vi "Auto-Pause Check.vi"(6 "Auto Stats":T1, 10 "Queue":refnum<queue>, 11 "Autopause":cluster{"GoodPause":u32, "RejectPause":u32}) -> (3 "Autopause out":cluster{"GoodPause":u32, "RejectPause":u32})   [LabVIEW 2021]
uses:
  support/Controls/Auto Stats.ctl
  RT/Controls/Auto Times.ctl
  support/Message Queue/Message Cluster.ctl
  support/Message Queue/Enqueue Message (Single).vi
  <vilib>/ErrorRing/Error Ring.xnode
  support/Message Queue/Message Queue.lvlib
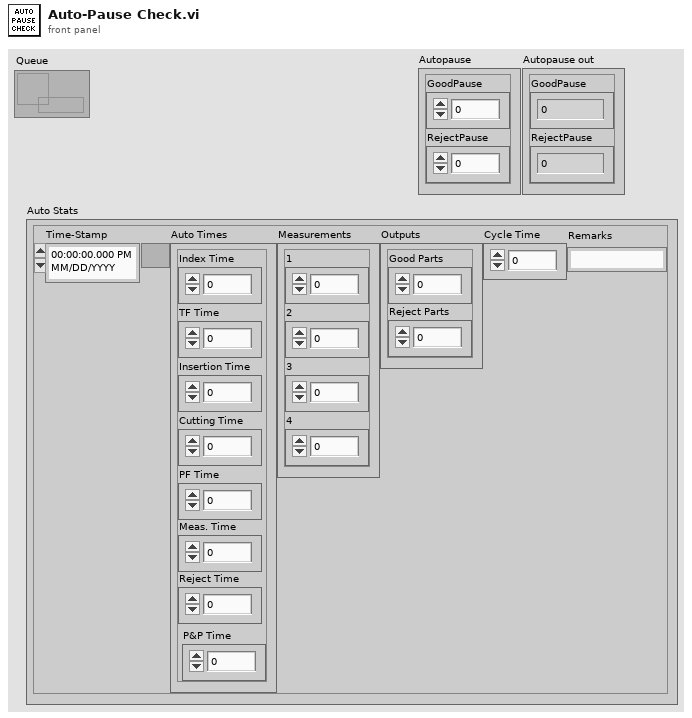
[diagram p1: front panel]
types:
  T1 = typedef "Auto Stats.ctl" = cluster{"Time-Stamp":timestamp, "Auto Times":T2, "Measurements":cluster{"1":dbl, "2":dbl, "3":dbl, "4":dbl}, "Outputs":cluster{"Good Parts":u32, "Reject Parts":u32}, "Cycle Time":dbl, "Remarks":string}
  T2 = typedef "Auto Times.ctl" = cluster{"Index Time":u32, "TF Time":u32, "Insertion Time":u32, "Cutting Time":u32, "PF Time":u32, "Meas. Time":u32, "Reject Time":u32, "P&P Time":u32}
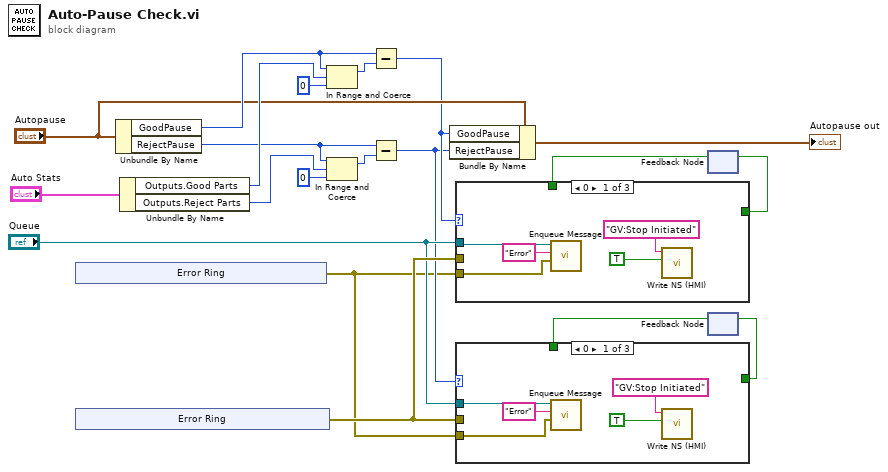
[diagram p0: block diagram]
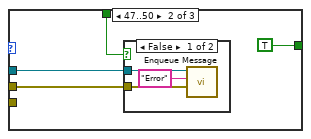
[diagram p2: hidden frame]
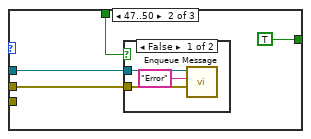
[diagram p5: hidden frame]
diagram:
  n1 = xnode "Error Ring"() -> ("error out"=w1:errorcluster)
  n2 = xnode "Error Ring"() -> ("error out"=w14:errorcluster)
  n3 = Unbundle By Name("Autopause") -> ("GoodPause"=w19:u32, "RejectPause"=w7:u32)
  n4 = Unbundle By Name("Auto Stats") -> ("Outputs.Good Parts"=w18:u32, "Outputs.Reject Parts"=w8:u32)
  n5 = In Range and Coerce(upper limit=w19, x=w18, lower limit=u32 0) -> (coerced(x)=w11:u32)  [unwired: 1 out]
  n6 = In Range and Coerce(upper limit=w7, x=w8, lower limit=u32 0) -> (coerced(x)=w10:u32)  [unwired: 1 out]
  n7 = Subtract(x=w19, y=w11) -> (x-y=w15:u32)
  n8 = Subtract(x=w7, y=w10) -> (x-y=w6:u32)
  n9 = Bundle By Name(cluster="Autopause", "GoodPause"=w15, "RejectPause"=w6) -> (→"Autopause out":cluster{"GoodPause":u32, "RejectPause":u32})
  n10 = feedback #1() -> (w4:bool)  [unwired: 1 in]
  n11 = case shown="0" w15 {
    tunnel: "Queue" -> [w22 w29 _]
    tunnel: w14 -> [_ w28 _]
    tunnel: [_ TRUE _] -> w5
    tunnel: w4 -> [_ w26 _]
    tunnel: w1 -> [w21 _ _]
    frame 0 {
      n12 = call-poly "Enqueue Message.vi"("Message Data"=w21, "Message"="Error", "Message Queue"=w22) -> ()  [unwired: 7 in, 2 out]
      n13 = call "Write NS (HMI).vi"("Message Data"=TRUE, "Message"="GV:Stop Initiated" ("string")) -> ()  [unwired: 9 in, 1 out]
    }
    frame 47..50 {
      n14 = case shown="False" w26 {
        tunnel: w29 -> [w31 _]
        tunnel: w28 -> [w30 _]
        frame False {
          n15 = call-poly "Enqueue Message.vi"("Message Data"=w30, "Message"="Error", "Message Queue"=w31) -> ()  [unwired: 7 in, 2 out]
        }
        frame True {
        }
      }
    }
    frame Default {
    }
  }
  n16 = feedback-in #1(w5) -> ()
  n17 = feedback #2() -> (w3:bool)  [unwired: 1 in]
  n18 = case shown="0" w6 {
    tunnel: "Queue" -> [w34 w41 _]
    tunnel: w14 -> [_ w40 _]
    tunnel: w3 -> [_ w39 _]
    tunnel: [_ TRUE _] -> w2
    tunnel: w1 -> [w33 _ _]
    frame 0 {
      n19 = call-poly "Enqueue Message.vi"("Message Data"=w33, "Message"="Error", "Message Queue"=w34) -> ()  [unwired: 7 in, 2 out]
      n20 = call "Write NS (HMI).vi"("Message Data"=TRUE, "Message"="GV:Stop Initiated" ("string")) -> ()  [unwired: 9 in, 1 out]
    }
    frame 47..50 {
      n21 = case shown="False" w39 {
        tunnel: w41 -> [w43 _]
        tunnel: w40 -> [w42 _]
        frame False {
          n22 = call-poly "Enqueue Message.vi"("Message Data"=w42, "Message"="Error", "Message Queue"=w43) -> ()  [unwired: 7 in, 2 out]
        }
        frame True {
        }
      }
    }
    frame Default {
    }
  }
  n23 = feedback-in #2(w2) -> ()
